vi "CAN Basic (FPGA).vi"(0 "Write CAN":bool, 1 "Transmit Frame":T2={"timestamp high"=0, "timestamp low"=0, "identifier"=5, "type"=enum."Data Frame", "info A"=0, "info B"=0, "data length"=8, "data"=[1, 2, 3, 4, 5, 6, 7, 8]} {"identifier" format="%x"; "timestamp high" format="%08x"; "timestamp low" format="%08x"; "data" format="%.0x"}) -> (2 "writing error":errorcluster)   [LabVIEW 2016]
doc: "This example demonstrates basic communication on the CAN bus. The example runs standalone (without a host VI).\n\nIt reads CAN frames on CAN 0 and displays a count along with the most recent frame. It transmits a CAN frame on CAN 1 each time you select the Transmit button. You can use the example simply by connecting a CAN cable (powered) between CAN 0 and CAN 1. To use the example with an external CAN device (such as an ECU), connect the device to CAN 0, then change the CAN Output node from CAN 1 to CAN 0. This enables you to interactively transmit and receive CAN frames with the external device.\n\nThis example assumes the following configuration for CAN 0 and CAN 1: Auto Start = True, Listen Only = False, Input Timeout = 10000ms, Output Timeout = 10000ms. The CAN Input and CAN Output nodes are configured to use Cluster for the CAN frame. For more information on configuration, refer to the Help for the NI 9852/9853 CAN module.\n\nIf you change this example such that the loops exit normally (such as a stop button), you must add the CAN Stop method to stop CAN communication before the VI stops execution. Only the LabVIEW abort button stops CAN communication when running standalone (no host VI).\n\nNote: Prior to running the VI, you will need to specify the VISA resource name for the FPGA target. You can specify the VISA resource name by right clicking the FPGA Target in the Project Explorer, then selecting Properties... and then specifying the VISA resource string."
uses:
  <vilib>/eio/EIONode/EIONode.xnode
  <vilib>/rvi/eio/common/nirviEmuTemplateMethod_errors.vi
  <vilib>/LabVIEW Targets/FPGA/RIO/nicrio_985x_controls.llb/CAN_IO_Frame Type.ctl
  <vilib>/LabVIEW Targets/FPGA/RIO/nicrio_985x_controls.llb/CAN_IO_Frame Cluster.ctl
  <vilib>/rvi/DataTransferAndStorage/Container/XNode/niFpgaContainer.xnode
  <vilib>/eio/EIOPropertyNode/EIOPropertyNode.xnode
  <vilib>/rvi/eio/common/nirviEmuTemplatePropertyGet_errors.vi
  <vilib>/rvi/eio/common/nirviEmuTemplatePropertyGet_noerrors.vi
  <vilib>/rvi/eio/common/nirviEmuTemplatePropertySet_errors.vi
  <vilib>/rvi/eio/common/nirviEmuTemplatePropertySet_noerrors.vi
  <vilib>/eio/EIOMethodNode/EIOMethodNode.xnode
  <vilib>/LabVIEW Targets/FPGA/RIO/nicrio_985x_controls.llb/CAN_IO_Comm State.ctl
  <vilib>/LabVIEW Targets/FPGA/RIO/nicrio_985x_controls.llb/CAN_IO_Frame Array U32.ctl
  <vilib>/rvi/FIFO/Fifo_Resource/nirvififoEmulationWrite.vi
panel:
  out "Frames Sent":u32
  in  "Reset CAN 0":bool
  out "CAN Comm State":T1
  out "error out":errorcluster
  out "9853 Serial Number":u32
  out "Frames lost?":bool
  out "Total Received":u32 format="%.0x"
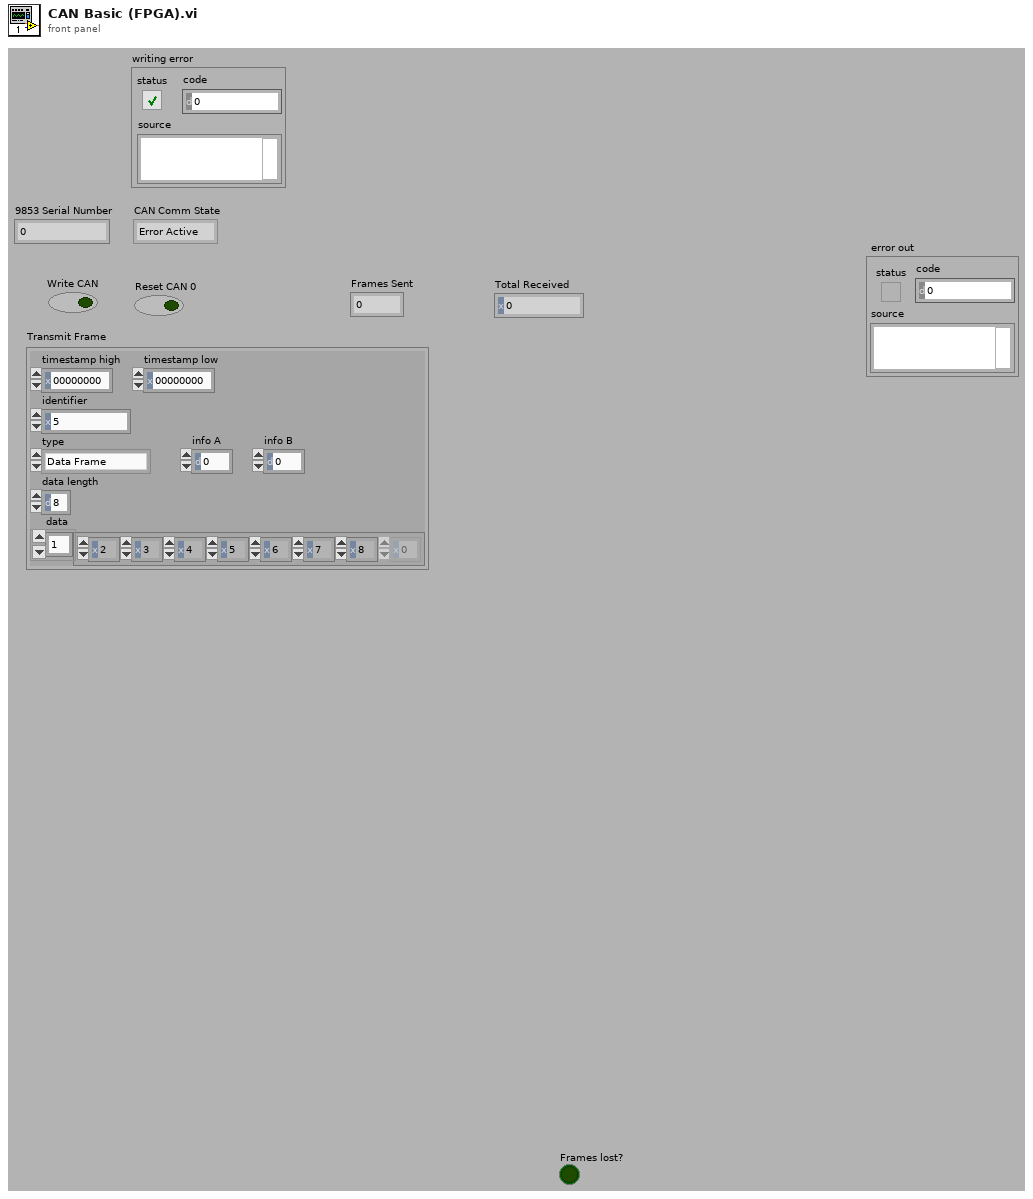
[diagram p1: front panel]
types:
  T1 = typedef "CAN_IO_Comm State.ctl" = enum8{"Error Active", "Error Passive", "Bus Off"}
  T2 = typedef "CAN_IO_Frame Cluster.ctl" = cluster{"timestamp high":u32, "timestamp low":u32, "identifier":u32, "type":T3, "info A":u8, "info B":u8, "data length":u8, "data":u8[]}
  T3 = typedef "CAN_IO_Frame Type.ctl" = enum8{"Data Frame", "Remote Frame", "(reserved)", "(reserved) ", "(reserved)  ", "(reserved)   ", "Bus Error", "Transceiver Fault"}
  T4 = typedef "CAN_IO_Frame Array U32.ctl" = u32[]
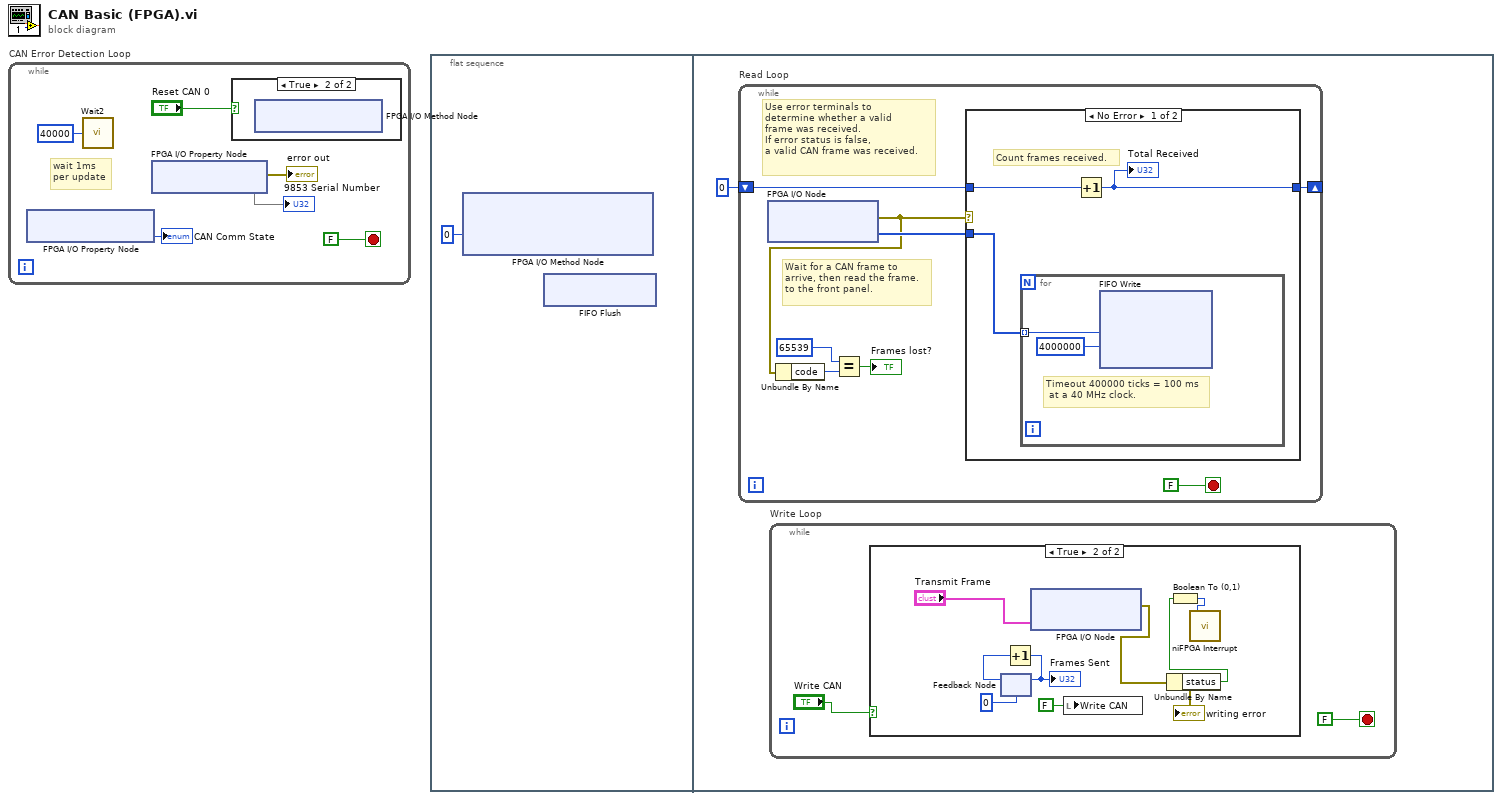
[diagram p0: block diagram]
diagram:
  n1 = while "CAN Error Detection Loop" {
    stop <- FALSE stop-if-true
    # "wait 1ms\nper update"
    n2 = xnode "FPGA I/O Property Node"() -> ("Comm State"=→"CAN Comm State":T1)  [unwired: 1 in, 1 out]
    n3 = call "Wait2"("Count(Ticks)"=u32 40000) -> ()  [unwired: 1 out]
    n4 = xnode "FPGA I/O Property Node"() -> ("error out"=→"error out":errorcluster, "Serial Number"=→"9853 Serial Number")  [unwired: 2 in, 1 out]
    n5 = case shown="True" "Reset CAN 0" {
      frame False {
      }
      frame True {
        n6 = xnode "FPGA I/O Method Node"() -> ()  [unwired: 1 in, 1 out]
      }
    }
  }
  n7 = flat-sequence {
    frame #0 {
      n8 = xnode "FPGA I/O Method Node"("Timeout"=0) -> ()  [unwired: 1 in, 2 out]
      n9 = xnode ("FIFO Flush")() -> ()  [unwired: 1 in, 1 out]
    }
    frame #1 {
      n10 = while "Read Loop" {
        shift-right: [w25] -> _
        shift-left: u32 0 ("Total Received") -> [w26]
        stop <- FALSE stop-if-true
        # "Use error terminals to \ndetermine whether a valid\nframe was received.  \nIf error status is false, \na valid CAN frame was received."
        # "Wait for a CAN frame to\narrive, then read the frame. \nto the front panel."
        n11 = xnode "FPGA I/O Node"() -> ("error out"=w19:errorcluster, "Mod1/CAN1"=w23:T4)  [unwired: 2 in, 1 out]
        n12 = Unbundle By Name(w19) -> ("code"=w20:i32)
        n13 = Equal?(x=65539, y=w20) -> (x = y?=→"Frames lost?":bool)
        n14 = case shown="No Error" w19 {
          tunnel: w23 -> [w27 _]
          tunnel: w26 -> [w29 w32]
          tunnel: [w28 w32] -> w25
          frame No Error {
            # "Count frames received."
            n15 = for {
              tunnel: w27 -> [w30] mode=indexing
              # "Timeout 400000 ticks = 100 ms\n at a 40 MHz clock."
              n16 = xnode ("FIFO Write")("Element"=w30, "Timeout"=4000000) -> ()  [unwired: 1 in, 2 out]
            }
            n17 = Increment(x=w29) -> (x+1=w28:u32)
            "Total Received" <- w28
          }
          frame Error {
          }
        }
      }
      n18 = while "Write Loop" {
        stop <- FALSE stop-if-true
        n19 = case shown="True" "Write CAN" {
          frame False {
          }
          frame True {
            n20 = feedback #1(u32 0) -> (w17:u32)
            n21 = Increment(x=w17) -> (x+1=w18:u32)
            "Frames Sent" <- w18
            n22 = feedback-in #1(w18) -> ()
            n23 = xnode "FPGA I/O Node"("Mod1/CAN1"="Transmit Frame") -> ("error out"=w13:errorcluster)  [unwired: 2 in, 1 out]
            "writing error" <- w13
            n24 = local write "Write CAN"(FALSE ("Write CAN")) -> ()
            n25 = Unbundle By Name(w13) -> ("status"=w12:bool)
            n26 = Boolean To (0,1)(Boolean=w12) -> (0, 1=w11:i16)
            n27 = call <vilib>:"niFPGA Interrupt.vi"("IRQ Number (0)"=w11) -> ()  [unwired: 2 in]
          }
        }
      }
    }
  }
